vi "MoveAnalysers.vi"(6 "Analysers Motor Control":T3=enum."Initialise & Get Angle", 8 "Interrupts on/off":bool=TRUE, 9 "file (use dialog)":path, 10 "Analysers Home to 45 Degrees":T1, 11 "Analyser Set Angles":cluster{"Analyser 1":i32, "Analyser 2":i32}) -> (1 "Analysers Moving?":T2, 2 "Found Home?":cluster{"Analyser 1":bool, "Analyser 2":bool}, 3 "Current Angles":cluster{"Analyser 1":i32, "Analyser 2":i32})   [LabVIEW 2014]
uses:
  typedef_analyser_motor_control.ctl
  Timer/typedef_timer.ctl
  Bool Crossing/typedef_twice_bool_crossing.ctl
panel:
  out "A2 Crenelation Interrupt State":i16(graph)
  out "A1 Crenelation Interrupt State":i16(graph)
  # "A1: True = +ve dir"
  # "A2: True = -ve dir"
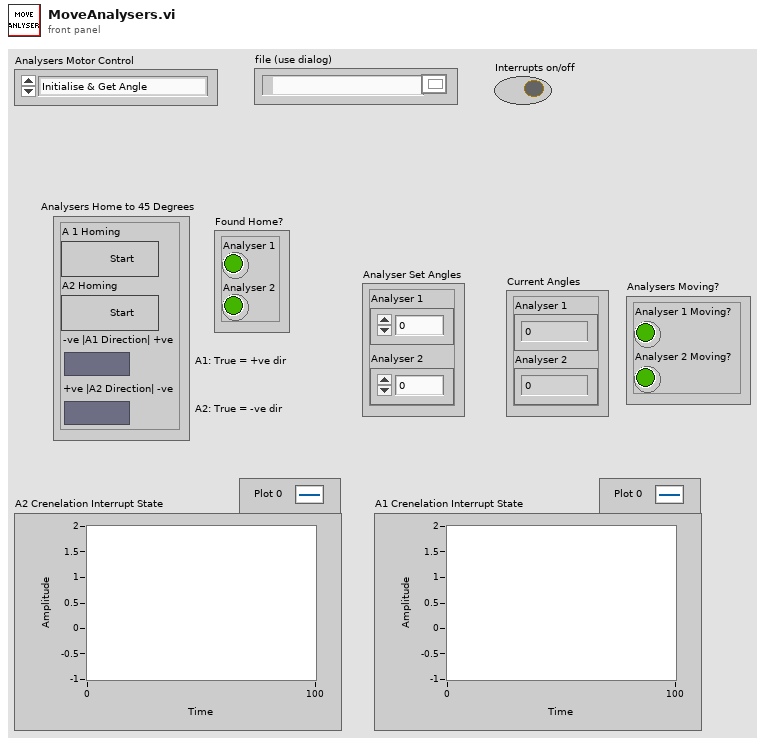
[diagram p1: front panel]
types:
  T1 = cluster{"A 1 Homing":bool, "A2 Homing ":bool, "-ve |A1 Direction| +ve":bool, "+ve |A2 Direction| -ve":bool}
  T2 = cluster{"Analyser 1 Moving?":bool, "Analyser 2 Moving?":bool}
  T3 = typedef "typedef_analyser_motor_control.ctl" = enum16{"Run", "Initialise & Get Angle", "Turn On/Off Interrupts", "Set Angle"}
  T4 = typedef "typedef_timer.ctl" = enum16{"Inside Time Window & Manual Reset", "Inside Time Window", "Reset", "Initialise", "Timed Out & Reset", "Timed Out"}
  T5 = typedef "typedef_twice_bool_crossing.ctl" = enum16{"F->T->F", "T->F->T", "Initialise"}
  T6 = cluster{"-ve |A1 Direction| +ve":bool, "+ve |A2 Direction| -ve":bool}
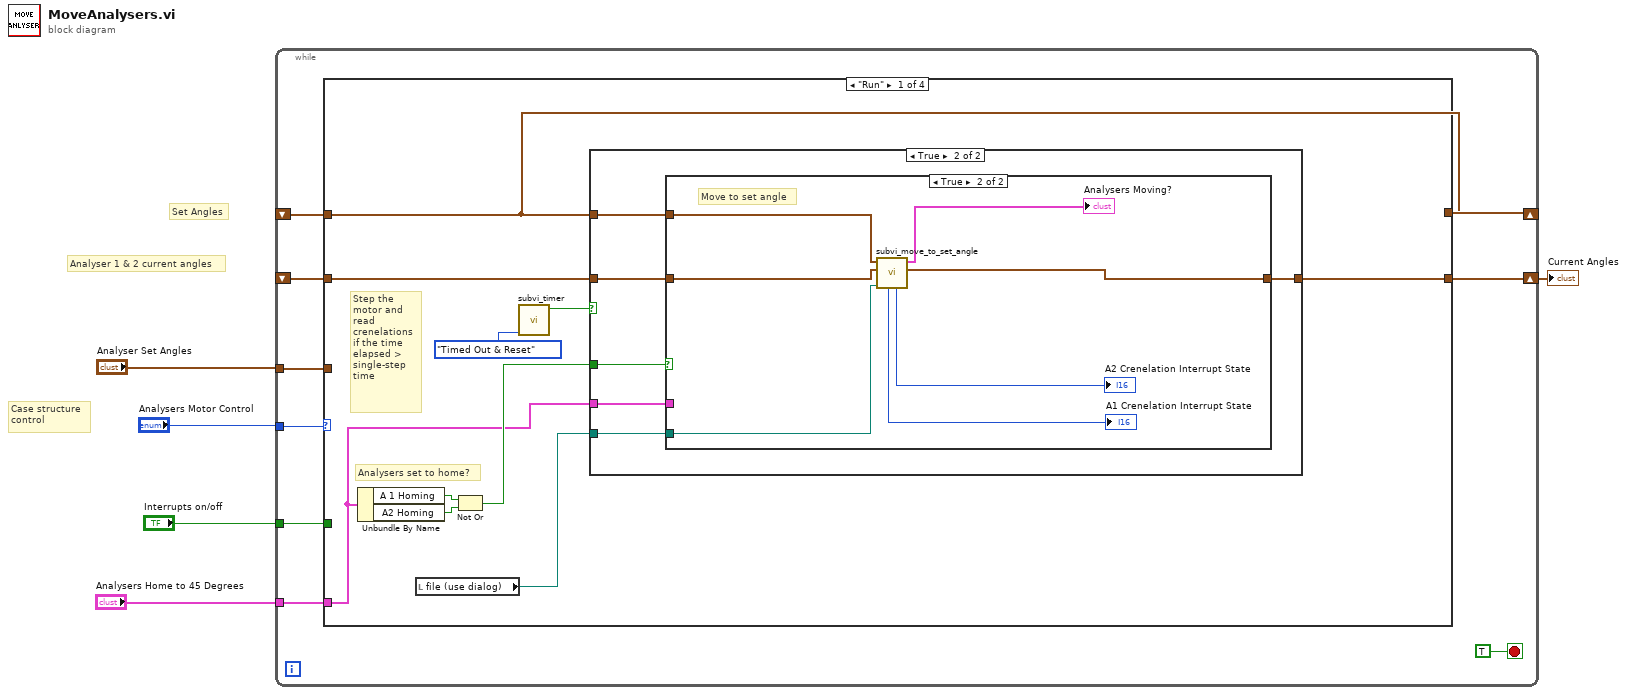
[diagram p0: block diagram]
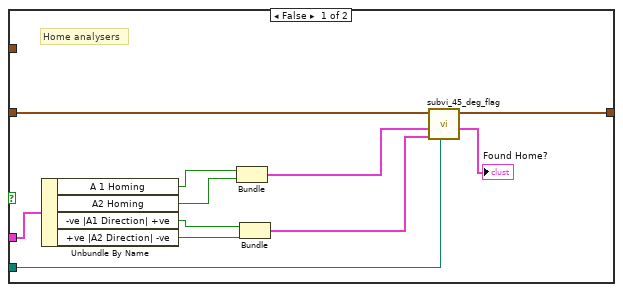
[diagram p3: hidden frame]
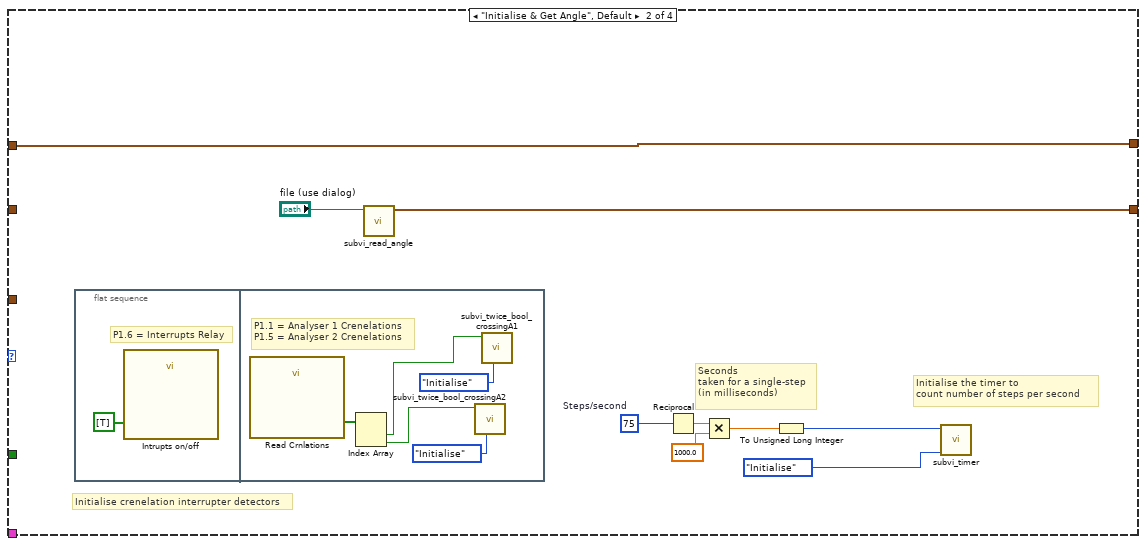
[diagram p4: hidden frame]
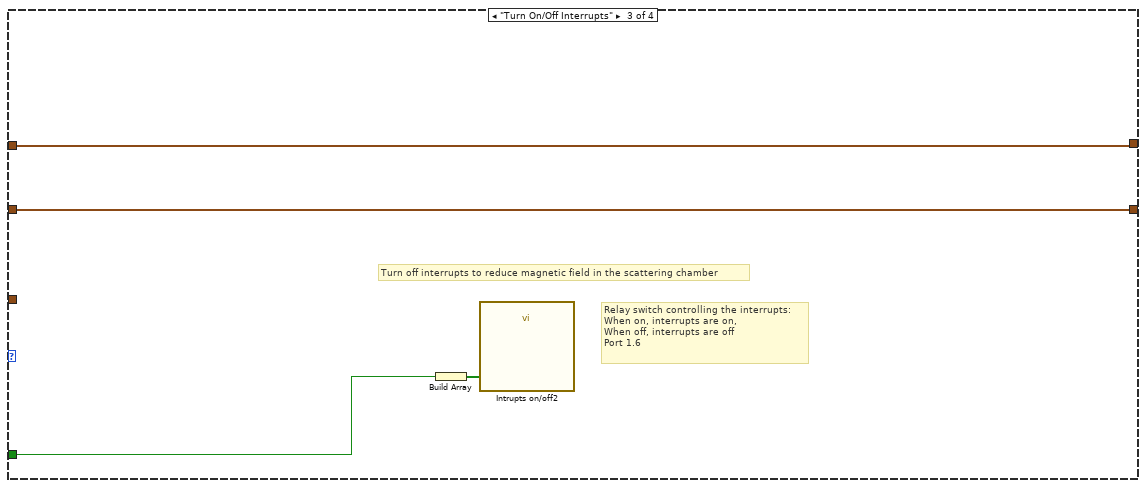
[diagram p5: hidden frame]
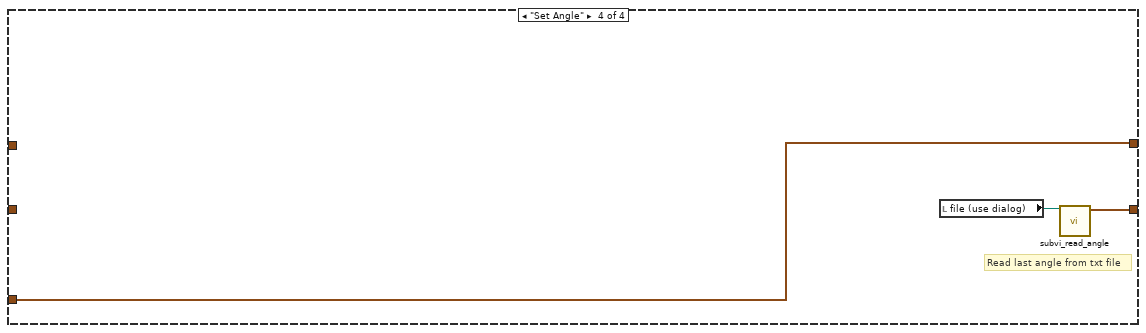
[diagram p6: hidden frame]
diagram:
  # "Set Angles"
  # "Analyser 1 & 2 current angles"
  # "Case structure \ncontrol"
  n1 = while {
    tunnel: "Analysers Motor Control" -> [w14]
    shift-right: [w13] -> w3
    shift-left: _ -> [w12]
    shift-right: [w9] -> _
    shift-left: _ -> [w11]
    tunnel: "Analyser Set Angles" -> [w8]
    tunnel: "Interrupts on/off" -> [w7]
    tunnel: "Analysers Home to 45 Degrees" -> [w6]
    stop <- TRUE stop-if-true
    n2 = case shown="\"Run\"" w14 {
      tunnel: [w19 w57 w68 w70] -> w13
      tunnel: w12 -> [w20 _ w68 _]
      tunnel: w11 -> [w21 w56 w67 _]
      tunnel: [w21 w56 w67 w71] -> w9
      tunnel: w8 -> [_ _ _ w71]
      tunnel: w7 -> [_ _ w65 _]
      tunnel: w6 -> [w15 _ _ _]
      frame "Run" {
        # "Analysers set to home?"
        # "Step the motor and read crenelations \nif the time elapsed > single-step time"
        n3 = Unbundle By Name(w15) -> ("A 1 Homing"=w18:bool, "A2 Homing"=w17:bool)
        n4 = local read "file (use dialog)"() -> (w22:path)
        n5 = Not Or(1:w17, 2:w18) -> (0:w16:bool)
        n6 = call "subvi_timer.vi"("Timer Functions"=typedef_timer."Timed Out & Reset") -> ("Timed Out?"=w23:bool)  [unwired: 9 in, 1 out]
        n7 = case shown="True" w23 {
          tunnel: w20 -> [w25 w27]
          tunnel: w21 -> [_ w31]
          tunnel: w22 -> [_ w29]
          tunnel: [w25 w30] -> w19
          tunnel: w16 -> [_ w28]
          tunnel: w15 -> [_ w26]
          frame False {
          }
          frame True {
            n8 = case shown="True" w28 {
              tunnel: w31 -> [_ w44]
              tunnel: [w42 w48] -> w30
              tunnel: w29 -> [w32 w45]
              tunnel: w27 -> [w41 w43]
              tunnel: w26 -> [w40 _]
              frame False {
                # "Home analysers"
                n9 = Unbundle By Name(w40) -> ("A 1 Homing"=w39:bool, "A2 Homing"=w38:bool, "-ve |A1 Direction| +ve"=w37:bool, "+ve |A2 Direction| -ve"=w36:bool)
                n10 = Bundle("A 1 Homing"=w39, "A2 Homing"=w38) -> (w35:cluster{"A 1 Homing":bool, "A2 Homing ":bool})  [unwired: 1 in]
                n11 = Bundle("-ve |A1 Direction| +ve"=w37, "+ve |A2 Direction| -ve"=w36) -> (w34:T6)  [unwired: 1 in]
                n12 = call "subvi_45_deg_flag.vi"("file (use dialog)"=w32, "Directions"=w34, "Analysers Moving?"=w35, "Current Angles"=w41) -> ("Found Home?"=→"Found Home?":cluster{"Analyser 1":bool, "Analyser 2":bool}, "New Current Angles"=w42:cluster{"Numeric Control":i32, "Analyser 2":i32})  [unwired: 6 in]
              }
              frame True {
                # "Move to set angle"
                n13 = call "subvi_move_to_set_angle.vi"("file (use dialog)"=w45, "Current Angles"=w43, "Analyser Set Angles"=w44) -> ("New Current Angles"=w48:cluster{"Analyser 1":i32, "Analyser 2":i32}, "Analysers Moving?"=→"Analysers Moving?":T2, "A2 Crenelation Interrupt State"=→"A2 Crenelation Interrupt State":i16, "A1 Crenelation Interrupt State"=→"A1 Crenelation Interrupt State":i16)  [unwired: 4 in, 1 out]
              }
            }
          }
        }
      }
      frame "Initialise & Get Angle", Default {
        w54 = 75  # Steps/second
        # "Initialise the timer to\ncount number of steps per second"
        # "Seconds \ntaken for a single-step\n(in milliseconds)"
        # "Initialise crenelation interrupter detectors"
        n14 = flat-sequence {
          frame #0 {
            # "P1.6 = Interrupts Relay"
            n15 = call "Intrupts on/off"("data"=bool[] [TRUE]) -> ()  [unwired: 17 in, 2 out]
          }
          frame #1 {
            # "P1.1 = Analyser 1 Crenelations\nP1.5 = Analyser 2 Crenelations"
            n16 = call "Read Crnlations"() -> ("data"=w62:bool[])  [unwired: 17 in, 2 out]
            n17 = Index Array(array=w62) -> (element #1=w61:bool, element #2=w60:bool)  [unwired: 2 in]
            n18 = call "subvi_twice_bool_crossingA2.vi"("Action"=typedef_twice_bool_crossing."Initialise", "Input Bool"=w60) -> ()  [unwired: 8 in, 2 out]
            n19 = call "subvi_twice_bool_crossingA1.vi"("Action"=typedef_twice_bool_crossing."Initialise", "Input Bool"=w61) -> ()  [unwired: 8 in, 2 out]
          }
        }
        n20 = call "subvi_read_angle.vi"("file (use dialog)"="file (use dialog)") -> ("Current Angles"=w57:cluster{"Analyser 1":i32, "Analyser 2":i32})  [unwired: 10 in]
        n21 = Reciprocal(x=w54) -> (1/x=w53:dbl)
        n22 = Multiply(x=w53, y=1000.0) -> (x*y=w51:dbl)
        n23 = To Unsigned Long Integer(number=w51) -> (unsigned 32bit integer=w50:u32)
        n24 = call "subvi_timer.vi"("Timer Functions"=typedef_timer."Initialise", "Threshold Time (ms)"=w50) -> ()  [unwired: 8 in, 2 out]
      }
      frame "Turn On/Off Interrupts" {
        # "Turn off interrupts to reduce magnetic field in the scattering chamber"
        # "Relay switch controlling the interrupts:\nWhen on, interrupts are on,\nWhen off, interrupts are off\nPort 1.6"
        n25 = Build Array(w65) -> (w66:bool[])
        n26 = call "Intrupts on/off2"("data"=w66) -> ()  [unwired: 17 in, 2 out]
      }
      frame "Set Angle" {
        # "Read last angle from txt file"
        n27 = local read "file (use dialog)"() -> (w69:path)
        n28 = call "subvi_read_angle.vi"("file (use dialog)"=w69) -> ("Current Angles"=w70:cluster{"Analyser 1":i32, "Analyser 2":i32})  [unwired: 10 in]
      }
    }
  }
  "Current Angles" <- w3
